vi "DiagnosticsToolKittest.vi"() -> ()   [LabVIEW 2010]
panel:
  out "Beta (0 official release, > 0 beta)":u32
  out "External Build":u32
  out "Minor Version":u32
  out "Major Version":u32
  out "Total Number of Devices":u32
  out "error out":errorcluster
  in  "error in (no error)":errorcluster
  # "DiagnosticsToolKitTest:\nRun this to find the number of available SITK(R) devices and current version.\nSITK(R) devices include the number of instruments found or defined (such as cameras\nor spectrometers) as well as internal devices available such as File and Calibration\nHandles.  If the number of devices is 0, verify that .r3x files are present in the\nLabVIEW folder (usually C:\\Program Files\\National Instruments\\LabVIEW x.x)."
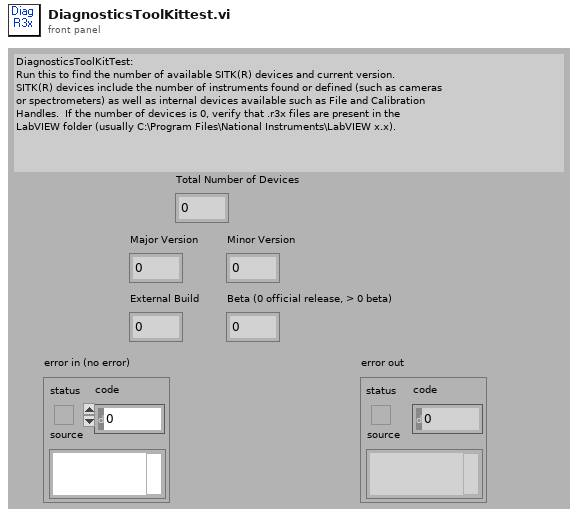
[diagram p1: front panel]
types:
  T1 = cluster{"Major Version":u32, "Minor Version":u32, "External Build":u32, "Internal Build":u32}
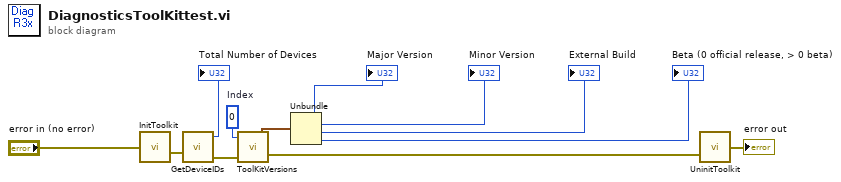
[diagram p0: block diagram]
diagram:
  w7 = 0  # Index
  n1 = call <userlib>:"InitToolkit.vi"("error in"="error in (no error)") -> ("error out"=w5:errorcluster)
  n2 = call <userlib>:"GetDeviceIDs.vi"("error in"=w5) -> ("Total Nuber of Devices or DLLs"=→"Total Number of Devices":u32, "error out"=w3:errorcluster)  [unwired: 1 in, 1 out]
  n3 = call <userlib>:"ToolKitVersions.vi"("error in"=w3, "Index"=w7) -> ("error out"=w2:errorcluster, "Versions"=w6:T1)  [unwired: 1 in, 1 out]
  n4 = Unbundle(w6) -> ("Major Version"=→"Major Version":u32, "Minor Version"=→"Minor Version":u32, "External Build"=→"External Build":u32, "Internal Build"=→"Beta (0 official release, > 0 beta)":u32)
  n5 = call <userlib>:"UninitToolkit.vi"("error in"=w2) -> ("error out"=→"error out":errorcluster)
